vi "CatchAndConvertInvalidImageTypes.vi"(0 "report in":refnum<class "NI_report.lvclass">, 5 "path to image":path, 9 "image format (jpeg)":enum32{"PNG", "JPEG", "GIF"}(ring)=enum."JPEG", 11 "error in (no error)":errorcluster) -> (4 "report out":refnum<class "NI_report.lvclass">, 6 "path to image out":path, 15 "error out":errorcluster)   [LabVIEW 2020, in "NI_report.lvclass"]
uses:
  NI_report.lvclass
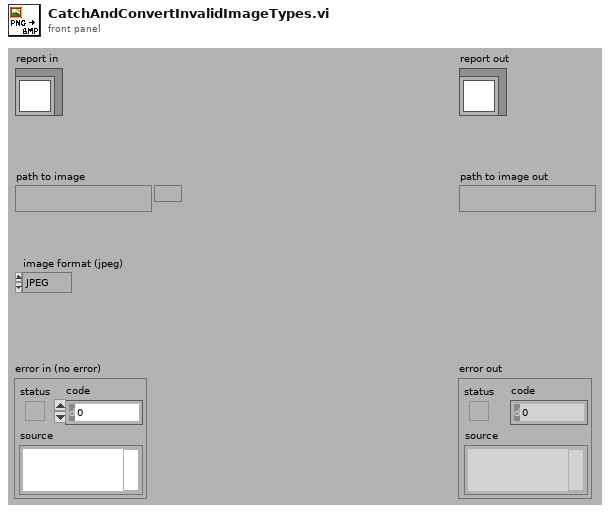
[diagram p1: front panel]
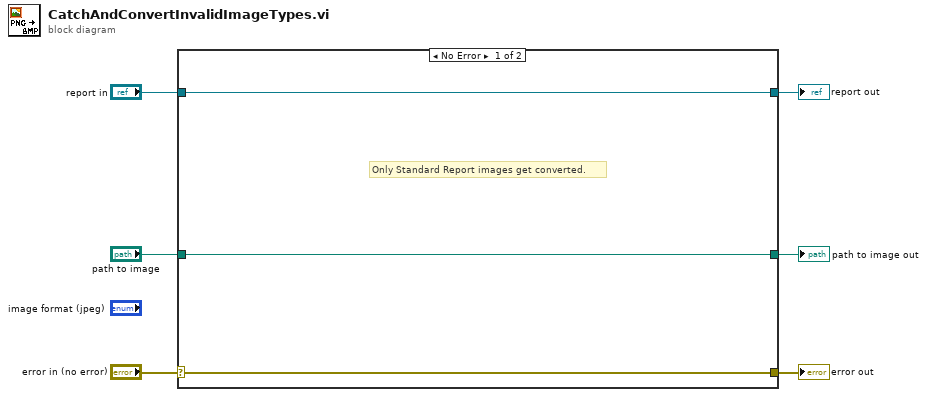
[diagram p0: block diagram]
diagram:
  n1 = case shown="No Error" "error in (no error)" {
    selector: "error in (no error)" -> [w8 w11]
    tunnel: [w8 w11] -> w5
    tunnel: [w9 w10] -> w3
    tunnel: "report in" -> [w9 w10]
    tunnel: "path to image" -> [w7 _]
    tunnel: [w7 _] -> w1
    frame No Error {
      # "Only Standard Report images get converted."
    }
    frame Error {
    }
  }
  "error out" <- w5
  "report out" <- w3
  "path to image out" <- w1
